vi "Read configuration.vi"(8 "error in":errorcluster, 11 "EthernetIP editor node in":refnum<class "EIP Tags editor node.lvclass">) -> (0 "error out":errorcluster, 2 "TBM configuration out":refnum<class "NISE_CEF_serializable configuration.lvclass">, 3 "EthernetIP editor node out":refnum<class "EIP Tags editor node.lvclass">)   [LabVIEW 2013, in "EIP Tags editor node.lvclass"]
uses:
  EIP Tags editor node.lvclass
  <vilib>/NI/Configuration Framework/serializable configuration/NISE_CEF_serializable configuration.lvclass
  EIP Tags editor node.lvclass/EIP Tags editor node.ctl
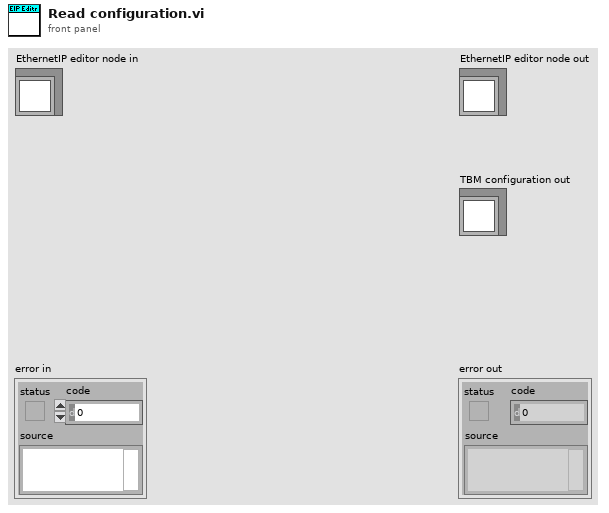
[diagram p1: front panel]
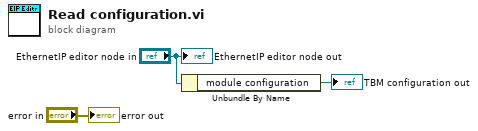
[diagram p0: block diagram]
diagram:
  n1 = Unbundle By Name("EthernetIP editor node in") -> ("module configuration"=→"TBM configuration out":refnum<class "EIP Tags Configuration.lvclass">)
  "error out" <- "error in"
  "EthernetIP editor node out" <- "EthernetIP editor node in"
